vi "Measurement_input_panel.vi"(0 "OK":T4, 2 "setup":T5, 5 "Setup filename":string) -> (11 "Setup filename out":string, 12 "Analysis Info cluster":T8[](array[typedef])=[{"Colour"=0, "Inst type"=enum."Pitot-static tube", "Inst name"="Manometer voltage", "Symbol"="U", "Code name"="", "Extra Info"="U", "Inst Array"=enum."PWA", "Extra Titles"=[], "Extra Values"=[], "U"=0.0, "u^2"=0.0, "u^3"=0.0, "u^4"=0.0, "Skew_u"=0.0, "Kurt_u"=0.0, "Sd Error in Mean"=0.0, "% u'/U"=0.0, "X"=0.0, "Y"=0.0, "Z"=0.0, "Timescale integral to 25%"=0.0, "Sd Error in Variance"=0.0, "Calib File"=path "", "Calib Constants"=[], "Output Position"=FALSE, "Full Stats"=FALSE, "Av Sampling Rate"=0.0, "Av No of Samples"=0.0, "Total Meas Time (s)"=0.0, "ADAM Ch Name"=""}, {"Colour"=0, "Inst type"=enum."Pitot-static tube", "Inst name"="Manometer voltage", "Symbol"="U", "Code name"="", "Extra Info"="U", "Inst Array"=enum."PWA", "Extra Titles"=[], "Extra Values"=[], "U"=0.0, "u^2"=0.0, "u^3"=0.0, "u^4"=0.0, "Skew_u"=0.0, "Kurt_u"=0.0, "Sd Error in Mean"=0.0, "% u'/U"=0.0, "X"=0.0, "Y"=0.0, "Z"=0.0, "Timescale integral to 25%"=0.0, "Sd Error in Variance"=0.0, "Calib File"=path "", "Calib Constants"=[], "Output Position"=FALSE, "Full Stats"=FALSE, "Av Sampling Rate"=0.0, "Av No of Samples"=0.0, "Total Meas Time (s)"=0.0, "ADAM Ch Name"=""}, {"Colour"=0, "Inst type"=enum."Pitot-static tube", "Inst name"="Manometer voltage", "Symbol"="U", "Code name"="", "Extra Info"="U", "Inst Array"=enum."PWA", "Extra Titles"=[], "Extra Values"=[], "U"=0.0, "u^2"=0.0, "u^3"=0.0, "u^4"=0.0, "Skew_u"=0.0, "Kurt_u"=0.0, "Sd Error in Mean"=0.0, "% u'/U"=0.0, "X"=0.0, "Y"=0.0, "Z"=0.0, "Timescale integral to 25%"=0.0, "Sd Error in Variance"=0.0, "Calib File"=path "", "Calib Constants"=[], "Output Position"=FALSE, "Full Stats"=FALSE, "Av Sampling Rate"=0.0, "Av No of Samples"=0.0, "Total Meas Time (s)"=0.0, "ADAM Ch Name"=""}] {"Sd Error in Variance" format="%.2f"; "Skew_u" format="%.2f"; "% u'/U" format="%.2f"; "Sd Error in Mean" format="%.2f"; "Kurt_u" format="%.2f"; "u^4" format="%.2f"; "u^3" format="%.2f"; "U" format="%.2f"; "u^2" format="%.2f"})   [LabVIEW 2013]
uses:
  Controls/Inst_type.ctl
  Controls/Analysis_info_cluster.ctl
  Controls/Instrument_Array.ctl
  Controls/LDA_Setup.ctl
  Controls/Setup.ctl
  Controls/ok_button.ctl
  Controls/Trigger_Mode.ctl
  Controls/PWA_Data.ctl
  File/Setup_Filetype.ctl
  Controls/Post_Process.ctl
  Controls/App_Global.ctl
  Controls/Ch_and_Spans.ctl
  Globals/Meas_global.vi
  Globals/Trav_pos_global.vi
  Globals/LDA_meas_global_1.vi
  Globals/Preference_global.vi
panel:
  in  "Acquisition Plug in":u16(ring) items=["ADAM_Server_Channels.vi", "DataTranslation.vi", "DT_With_Multiplexer.vi", "LDA_IP.vi", "NI-DAQmx.vi", "Simulate_kernal.vi"]
  in  "Select Duplicate Channels":bool
  in  "PWA Data":T1
  out "Inst type":T2
  in  "Edit temp and Press":bool
  out "Abs Press (mbar)":dbl=1013.0 format="%.1f"
  out "Temp (deg C)":dbl=21.0 format="%.1f"
  in  "Trigger mode":T3
  in  "Select Plug Ins":bool
  in  "Sync Delay Time (ms)":dbl=24.0 format="%.2f"
  out "XW Present?":bool
  out "Read Setup File?":bool
  out "Setup Paths":string[](array[string])
  in  "Select ADAM Channels":bool
  in  "stop":bool
  out "Notes":string
  in  "Setup filename selector":u16(ring) items=["Current_Setup.xls", "Copy of Current_Setup.xls", "thermistor-rake.xls", "Current_Setup.xls", "thermistor-rake.xls"]
  in  "Synchronise Analogue channels with LDA":bool
  in  "LDA set up":T6={"dimensions"=enum."2D", "Analogue Freq Multiplier"=0.1} {"Analogue Freq Multiplier" min=0.1 max=100.0 format="%_5g"}
  in  "LDA data":enum16{"No LDA data", "Take LDA data"}(ring)=enum."Take LDA data"
  in  "Cross wire":T7(ring)
  in  "No of Analogue inst":i32=1
  in  "Ch & spans choices":T10(array[cluster]) {"D" format="%.2f"; "Ch No" min=0; "low limit" min=-10 max=10 format="%.2f"; "high limit" min=-10 max=10 format="%.2f"}
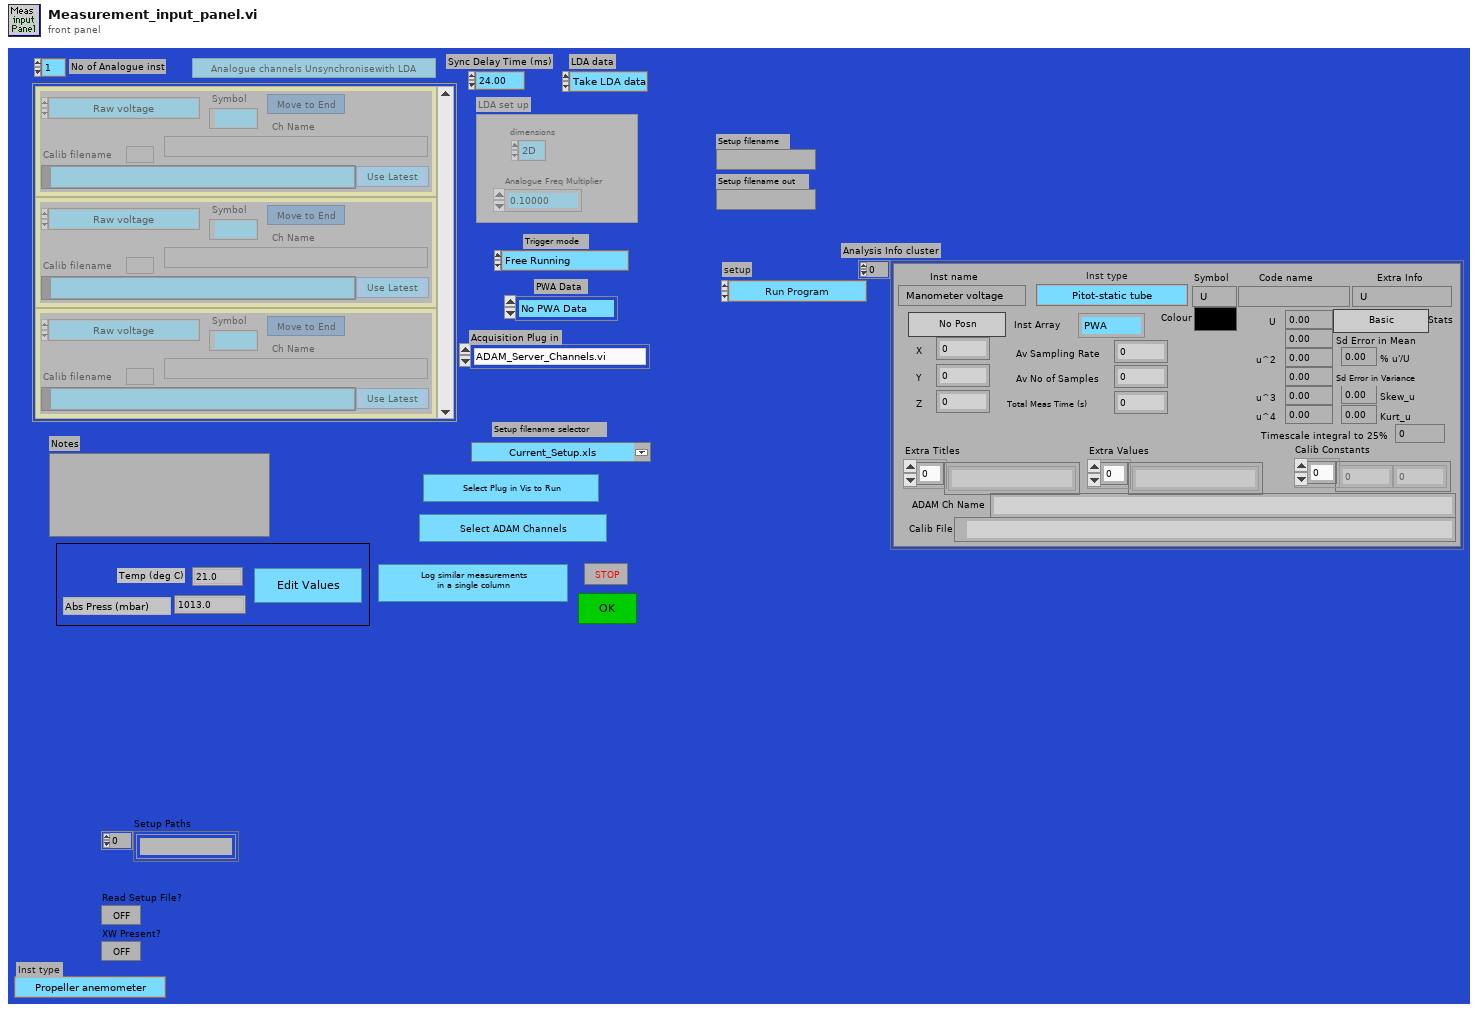
[diagram p1: front panel]
types:
  T1 = typedef "PWA_Data.ctl" = enum16{"No PWA Data", "One Ch PWA"}
  T2 = typedef "Inst_type.ctl" = enum16{"Propeller anemometer", "Raw voltage", "Pressure Transducer", "Pitot-static tube", "Preston tube", "Hot wire", "Cross wire 1", "Cross wire 2", "Generic Linear", "Generic Polynomial", "Generic BackPoly", "Fast FID", "Thermocouple", "Cold wire", "Pulsed Wire", "LDA Vel", "LDA Tran time", "LDA Arr time"}
  T3 = typedef "Trigger_Mode.ctl" = enum16{"Free Running", "Start on Trigger", "Trigger Every Block", "Trigger Every Sample"}
  T4 = typedef "ok_button.ctl" = bool
  T5 = typedef "Setup.ctl" = enum16{"Run Program", "Show Setup", "Save Current Setup", "Setup Front Panel"}
  T6 = typedef "LDA_Setup.ctl" = cluster{"dimensions":enum16{"1D", "2D"}, "Analogue Freq Multiplier":dbl}
  T7 = enum16{"2nd component as calculated", "2nd component multipled by -1"}
  T8 = typedef "Analysis_info_cluster.ctl" = cluster{"Colour":u32, "Inst type":T2, "Inst name":string, "Symbol":string, "Code name":string, "Extra Info":string, "Inst Array":T9, "Extra Titles":string[], "Extra Values":string[], "U":dbl, "u^2":dbl, "u^3":dbl, "u^4":dbl, "Skew_u":dbl, "Kurt_u":dbl, "Sd Error in Mean":dbl, "% u'/U":dbl, "X":dbl, "Y":dbl, "Z":dbl, "Timescale integral to 25%":dbl, "Sd Error in Variance":dbl, "Calib File":path, "Calib Constants":dbl[], "Output Position":bool, "Full Stats":bool, "Av Sampling Rate":dbl, "Av No of Samples":dbl, "Total Meas Time (s)":dbl, "ADAM Ch Name":string}
  T9 = typedef "Instrument_Array.ctl" = enum16{"PWA", "LDA", "Analogue"}
  T10 = cluster{"high limit":sgl, "low limit":sgl, "Ch No":i16, "Calib filename":path, "Inst type":T2, "Symbol":string, "Move channel":bool, "Use Latest":bool, "D":dbl, "Ch Name":string}[]
  T11 = typedef "Post_Process.ctl" = enum16{"Take New Data", "Post Process Raw Data File"}
  T12 = typedef "Setup_Filetype.ctl" = enum16{"Measurement Setups", "Calibration Setups", "General", "Results File Plotter Setups", "Speed Calib Tweaks"}
  T13 = typedef "App_Global.ctl" = enum16{"Read Global", "Write to Global", "Initialise Array"}
  T14 = typedef "Ch_and_Spans.ctl" = cluster{"high limit (10V)":sgl, "low limit (-10V)":sgl, "Ch No":i16, "Var name":string, "Use Latest Calib":bool}
  T15 = enum16{"Zero or one", "One", "Zero or more", "One or more"}
  T16 = typedef "Traverse_cluster.ctl" = cluster{"Start X":dbl, "Start Y":dbl, "Start Z":dbl, "End X":dbl, "End Y":dbl, "End Z":dbl, "No. of pts.":i32, "Spacing":T17, "Filename":path, "Tunnel Speed":dbl, "Averaging time (min)":dbl, "Extra Commands":string, "Specific Arguments":string, "Emission Rate (l/min)":dbl, "Trace Gas Concentration (%)":dbl, "Density Ratio":string, "Comments":string, "Row No":i32, "Row Type Selector":T18, "Completion time":string, "Row Duration (mins)":dbl, "No. of Valid pts.":i32, "Meas Setup File":string}
  T17 = typedef "Spacing.ctl" = enum16{"Linear", "Log", "Gauss", "Specified", "N/A"}
  T18 = typedef "Multi_run_mode.ctl" = enum16{"Move Traverse Only", "Set Tunnel Speed Only", "Set Source Only", "Set Measurement Conditions", "Single Measurement", "Vertical Profile", "Lateral Profile", "Longitudinal Profile", "Explore Volume", "Multi-Axis Profile", "Auto Calibrate", "Meas Fast FID Bkgnd", "Check Beam Power", "Scanning Valve Measurement", "Run VI Named:", "Set ADAM Ch", "Wait (minutes)", "Send Message", "Synchronize With:", "Fall Back to this Row", "Turn Off Row Repeating", "Blank Row", "Traverse 3D Volume"}
  T19 = cluster{"high limit (10V)":sgl, "low limit (-10V)":sgl, "Ch No":i16, "Calib filename":path, "Inst type":T2, "Symbol":string, "Move channel":bool, "Use Latest":bool, "D":dbl, "Ch Name":string}[]
  T20 = cluster{"high limit":sgl, "low limit":sgl, "Ch No":i16, "Calib filename":path, "Inst type":T2, "Symbol":string, "Move channel":bool, "Use Latest":bool, "D":dbl, "Ch Name":string}
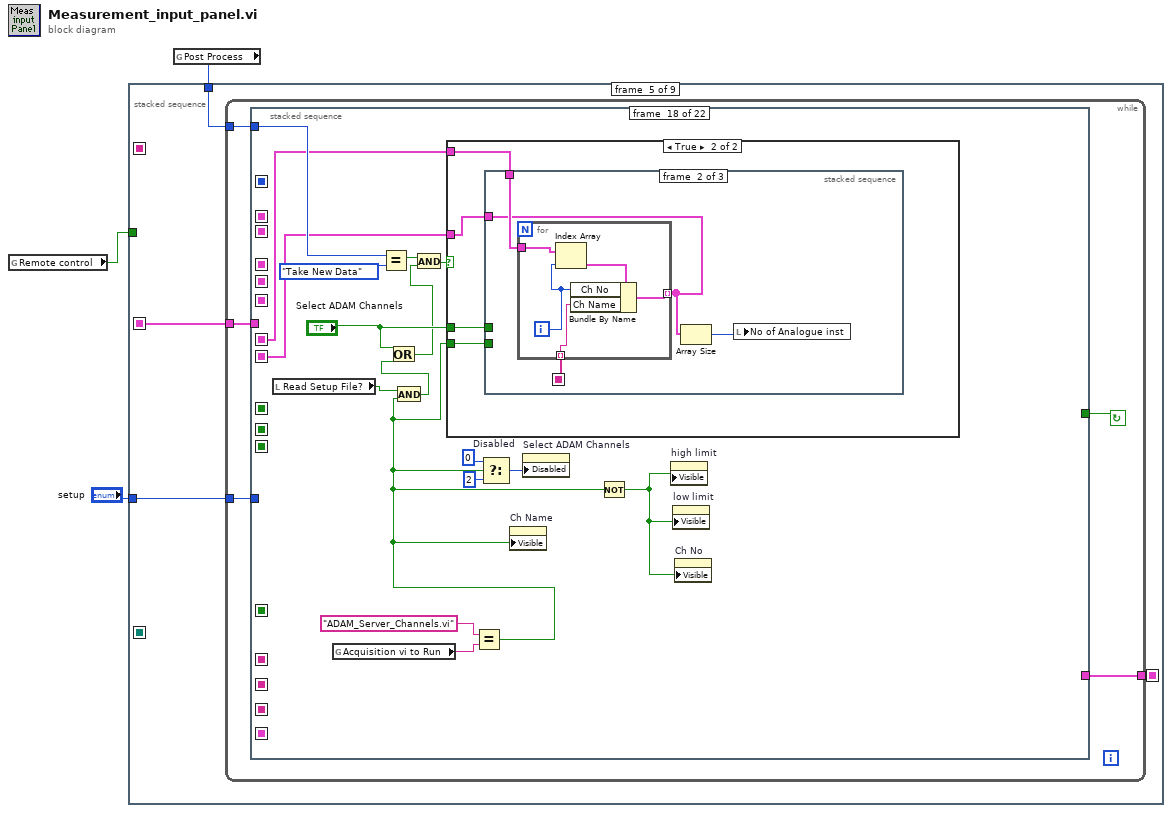
[diagram p0: block diagram]
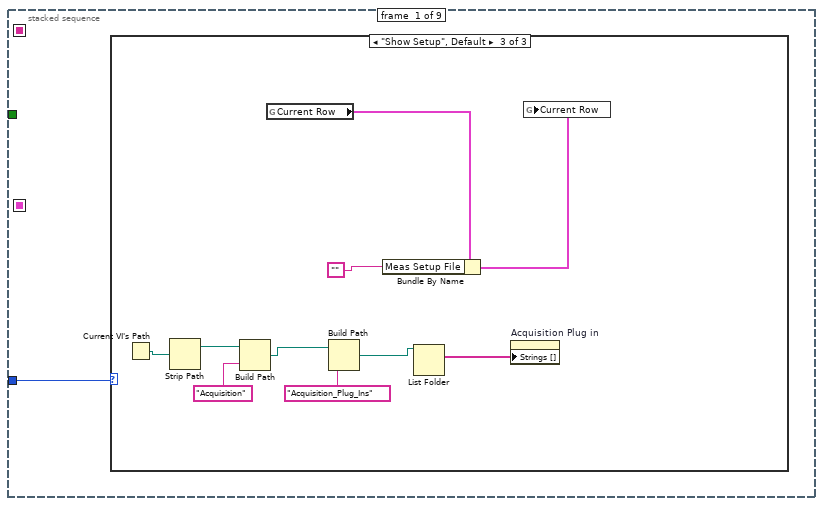
[diagram p2: hidden frame]
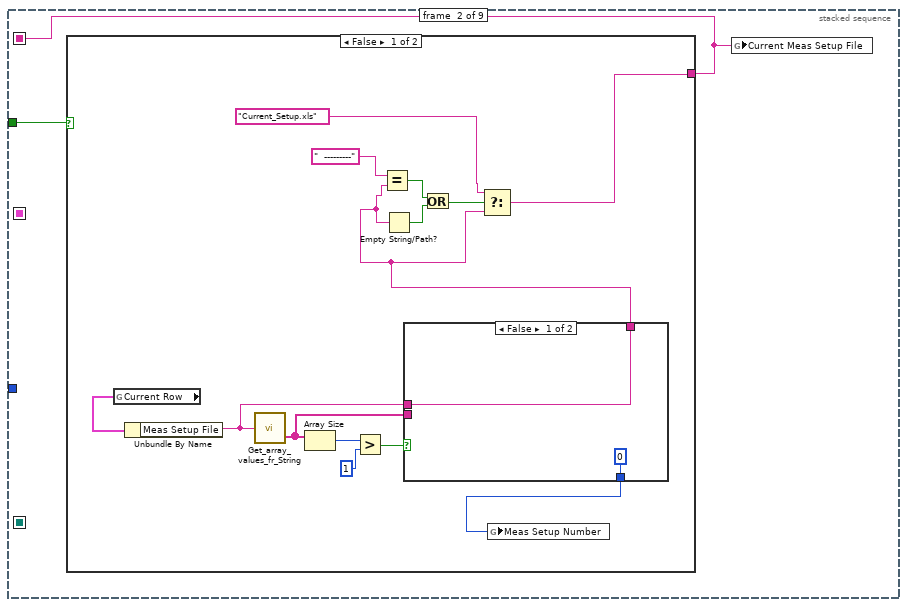
[diagram p5: hidden frame]
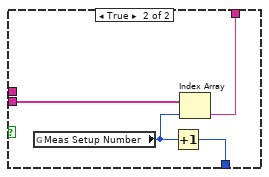
[diagram p6: hidden frame]
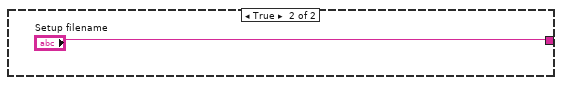
[diagram p7: hidden frame]
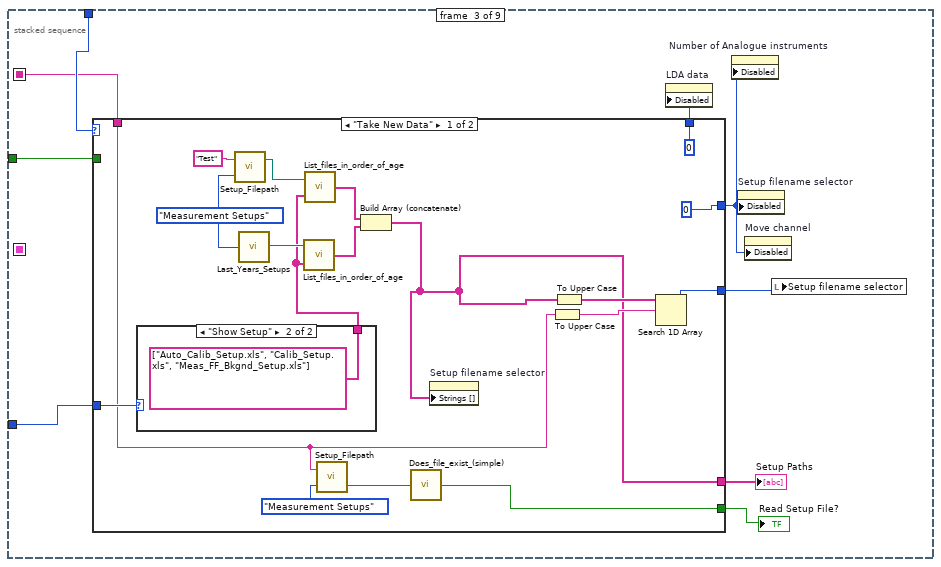
[diagram p8: hidden frame]
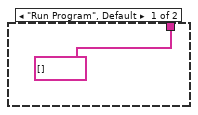
[diagram p9: hidden frame]
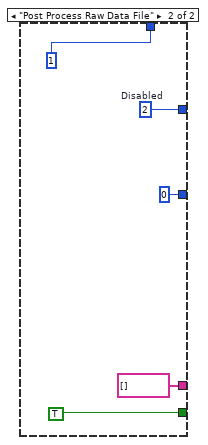
[diagram p10: hidden frame]
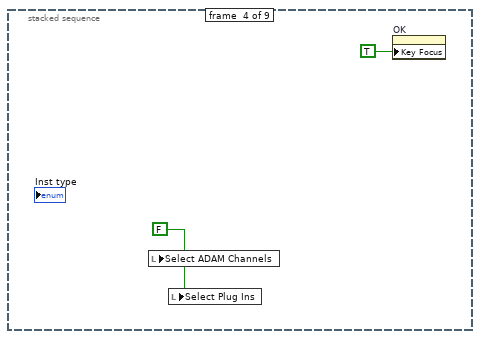
[diagram p11: hidden frame]
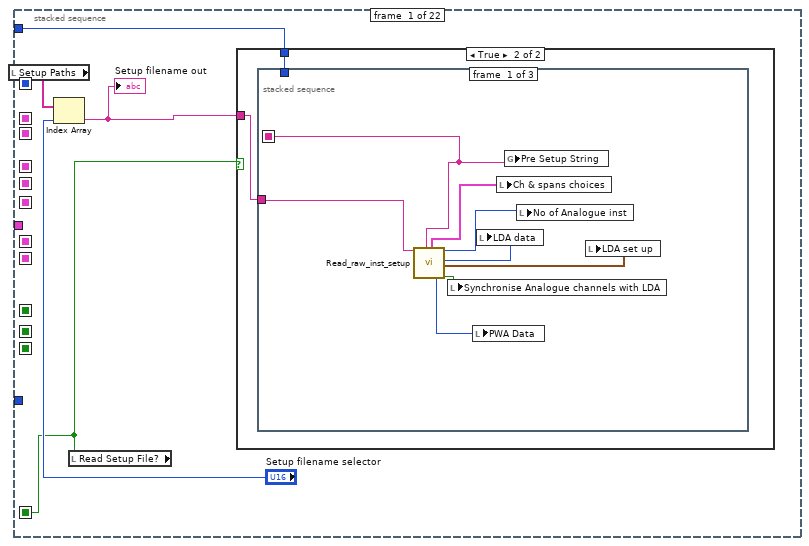
[diagram p12: hidden frame]
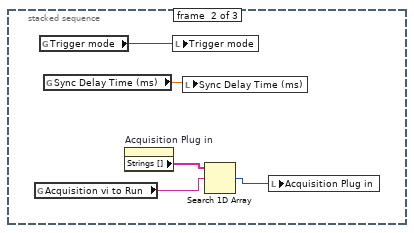
[diagram p14: hidden frame]
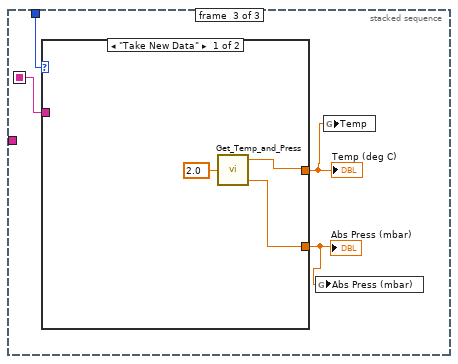
[diagram p15: hidden frame]
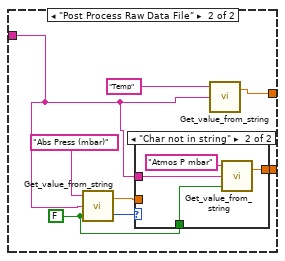
[diagram p16: hidden frame]
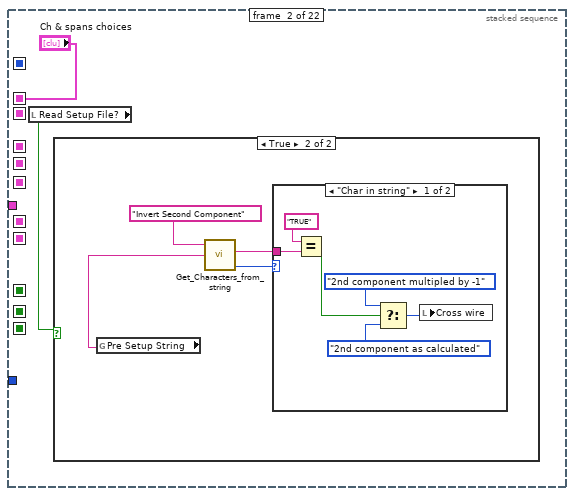
[diagram p18: hidden frame]
diagram:
  n1 = global read "Meas_global.vi" "Remote control"() -> (w1:bool)
  n2 = global read "Meas_global.vi" "Post Process"() -> (w3:T11)
  n3 = stacked-sequence {
    seq-local: [_ _ _ _ w77 _ _ _ _] -> [_ _ _ _ _ _ w694 w795 _]
    seq-local: [_ w15 _ _ _ _ _ _ _] -> [_ _ w38 _ _ _ w693 _ _]
    seq-local: [_ _ _ _ w74 _ _ _ _] -> [_ _ _ _ _ _ _ _ w847]
    seq-local: [_ _ _ _ _ _ _ w794 _] -> [_ _ _ _ _ _ _ _ w846]
    tunnel: w3 -> [_ _ w46 _ w76 _ _ w796 _]
    tunnel: "setup" -> [w4 _ w40 _ w75 _ w695 _ _]
    tunnel: w1 -> [_ w16 w39 _ _ _ _ _ _]
    frame #0 {
      n4 = case shown="\"Show Setup\", Default" w4 {
        frame "Run Program" {
        }
        frame "Setup Front Panel" {
        }
        frame "Show Setup", Default {
          n5 = Current VI's Path() -> (path=w11:path)
          n6 = Strip Path(path=w11) -> (stripped path=w10:path)  [unwired: 1 out]
          n7 = Build Path(base path=w10, name or relative path="Acquisition") -> (appended path=w7:path)
          n8 = global read "Trav_pos_global.vi" "Current Row"() -> (w14:T16)
          n9 = Build Path(base path=w7, name or relative path="Acquisition_Plug_Ins") -> (appended path=w6:path)
          n10 = Bundle By Name(cluster=w14, "Meas Setup File"="") -> (w13:T16)
          n11 = List Folder(path=w6) -> (filenames=w5:string[])  [unwired: 3 in, 3 out]
          n12 = property on="Acquisition Plug in" class="Ring (strict)"("Strings []"=w5) -> ()  [unwired: 2 in, 2 out]
          n13 = global write "Trav_pos_global.vi" "Current Row"(w13) -> ()
        }
      }
    }
    frame #1 {
      n14 = case shown="False" w16 {
        tunnel: [w29 "Setup filename"] -> w15
        frame False {
          n15 = global read "Trav_pos_global.vi" "Current Row"() -> (w25:T16)
          n16 = Unbundle By Name(w25) -> ("Meas Setup File"=w19:string)
          n17 = call "Get_array_values_fr_String.vi"("String Value"=w19) -> ("String array"=w18:string[])  [unwired: 1 out]
          n18 = Array Size(array=w18) -> (size(s)=w23:i32)
          n19 = Greater?(x=w23, y=1) -> (0:w21:bool)
          n20 = case shown="False" w21 {
            tunnel: [w32 w35] -> w20
            tunnel: w19 -> [w32 _]
            tunnel: w18 -> [_ w36]
            tunnel: [0 w33] -> w17
            frame False {
            }
            frame True {
              n21 = global read "Trav_pos_global.vi" "Meas Setup Number"() -> (w34:i32)
              n22 = Increment(x=w34) -> (x+1=w33:i32)
              n23 = Index Array(array=w36, index=w34) -> (element=w35:string)
            }
          }
          n24 = Equal?(x="  ---------" ("f"), y=w20) -> (x = y?=w28:bool)
          n25 = Empty String/Path?(string/path=w20) -> (empty?=w27:bool)
          n26 = Or(x=w28, y=w27) -> (x .or. y?=w24:bool)
          n27 = Select(t="Current_Setup.xls", s=w24, f=w20) -> (s? t:f=w29:string)
          n28 = global write "Trav_pos_global.vi" "Meas Setup Number"(w17) -> ()
        }
        frame True {
        }
      }
      n29 = global write "Trav_pos_global.vi" "Current Meas Setup File"(w15) -> ()
    }
    frame #2 {
      n30 = case shown="\"Take New Data\"" w46 {
        tunnel: [w47 string[] []] -> w42
        tunnel: [w60 TRUE ("exists")] -> w41
        tunnel: [u8 0 ("Disabled") w68] -> w43
        tunnel: [u8 0 ("Disabled") u8 1 ("Disabled")] -> w45
        tunnel: w38 -> [w56 _]
        tunnel: [w63 0 ("index of element")] -> w44
        tunnel: w40 -> [w58 _]
        tunnel: w39 -> [_ _]
        frame "Take New Data" {
          w50 = Setup_Filetype."Measurement Setups" ("Setup File Type")
          n31 = case shown="\"Show Setup\"" w58 {
            tunnel: [string[] [] ("file names") string[] ["Auto_Calib_Setup.xls", "Calib_Setup.xls", "Meas_FF_Bkgnd_Setup.xls"] ("file names")] -> w48
            frame "Run Program", Default {
            }
            frame "Show Setup" {
            }
          }
          n32 = call "Setup_Filepath.vi"("Setup File Type"=w50, "Filename in"="Test") -> ("Directory"=w51:path)  [unwired: 1 out]
          n33 = call "Last_Years_Setups.vi"("Setup File Type"=w50) -> ("Directory"=w49:path)
          n34 = call "List_files_in_order_of_age.vi"("Files to Hide"=w48, "Folder"=w49) -> ("file names"=w53:string[])
          n35 = call "List_files_in_order_of_age.vi"("Files to Hide"=w48, "Folder"=w51) -> ("file names"=w52:string[])
          n36 = call "Setup_Filepath.vi"("Setup File Type"=Setup_Filetype."Measurement Setups", "Filename in"=w56) -> ("Filename Out"=w55:path)  [unwired: 1 out]
          n37 = Build Array (concatenate)(w52, w53) -> (w47:string[])
          n38 = call "Does_file_exist_(simple).vi"("Pathname"=w55) -> ("exists?"=w60:bool)
          n39 = property on="Setup filename selector" class="Ring (strict)"("Strings []"=w47) -> ()  [unwired: 2 in, 2 out]
          n40 = To Upper Case(1:w56) -> (0:w61:string)
          n41 = To Upper Case(1:w47) -> (0:w62:string[])
          n42 = Search 1D Array(1D array=w62, element=w61) -> (index of element=w63:i32)  [unwired: 1 out]
        }
        frame "Post Process Raw Data File" {
          w68 = u8 2  # Disabled
        }
      }
      "Setup Paths" <- w42
      "Read Setup File?" <- w41
      n43 = property on="LDA data" class="Enum (strict)"("Disabled"=w45) -> ()  [unwired: 2 in, 2 out]
      n44 = property on="Number of Analogue instruments" class="DigNum (strict)"("Disabled"=w43) -> ()  [unwired: 2 in, 2 out]
      n45 = property on="Setup filename selector" class="Ring (strict)"("Disabled"=w43) -> ()  [unwired: 2 in, 2 out]
      n46 = property on="Move channel" class="Bool (strict)"("Disabled"=w43) -> ()  [unwired: 2 in, 2 out]
      n47 = local write "Setup filename selector"(w44) -> ()
    }
    frame #3 {
      w73 = FALSE ("Select Local ADAM Channels")
      n48 = local write "Select ADAM Channels"(w73) -> ()
      n49 = local write "Select Plug Ins"(w73) -> ()
      n50 = property on="OK" class="Bool"("Key Focus"=TRUE) -> ()  [unwired: 2 in, 2 out]
    }
    frame #4 {
      n51 = while {
        tunnel: w75 -> [w79]
        tunnel: w76 -> [w80]
        tunnel: [w82] -> w77
        tunnel: [w78] -> w74
        stop <- w81 continue-if-true
        n52 = stacked-sequence {
          seq-local: [_ _ _ _ _ _ _ _ w198 _ _ _ _ _ _ _ _ _ _ _ _ _] -> [_ _ _ _ _ _ _ _ _ _ w261 w306 w351 _ _ _ _ _ _ _ _ _]
          seq-local: [_ "Ch & spans choices" _ _ _ _ _ _ _ _ _ _ _ _ _ _ _ _ _ _ _ _] -> [_ _ _ _ _ w160 _ w194 w199 _ _ _ _ _ _ _ _ _ w579 _ _ _]
          seq-local: [_ _ _ _ _ w165 _ _ _ _ _ _ _ _ _ _ _ _ _ _ _ _] -> [_ _ _ _ _ _ _ _ w200 _ _ _ _ _ _ _ _ _ _ _ _ _]
          seq-local: [_ _ _ _ _ _ _ _ _ _ w263 _ _ _ _ _ _ _ _ _ _ _] -> [_ _ _ _ _ _ _ _ _ _ _ w308 _ _ _ _ _ _ _ _ _ w659]
          seq-local: [_ _ _ _ _ _ _ _ _ _ _ _ _ w384 _ _ _ _ _ _ _ _] -> [_ _ _ _ _ _ _ _ _ _ _ _ _ _ w403 _ _ _ _ _ _ _]
          seq-local: [_ _ _ _ _ _ _ _ _ _ _ _ _ _ w399 _ _ _ _ _ _ _] -> [_ _ _ _ _ _ _ _ _ _ _ _ _ _ _ w427 w493 _ _ _ w635 w660]
          seq-local: [_ _ _ _ _ _ _ _ _ _ _ w312 _ _ _ _ _ _ _ _ _ _] -> [_ _ _ _ _ _ _ _ _ _ _ _ _ w381 _ _ _ _ _ _ _ _]
          seq-local: [_ _ _ _ _ _ _ _ _ _ _ _ w355 _ _ _ _ _ _ _ _ _] -> [_ _ _ _ _ _ _ _ _ _ _ _ _ w380 _ _ _ _ _ _ _ _]
          seq-local: [_ _ _ _ _ _ _ _ _ w258 _ _ _ _ _ _ _ _ _ _ _ _] -> [_ _ _ _ _ _ _ _ _ _ w262 w309 _ _ _ _ _ _ _ _ _ w658]
          seq-local: [_ _ _ _ _ _ _ _ _ _ _ _ _ _ _ w426 _ _ _ _ _ _] -> [_ _ _ _ _ _ _ _ _ _ _ _ _ _ _ _ w496 _ _ _ _ _]
          seq-local: [_ _ _ _ _ _ _ _ _ _ _ _ _ _ _ w425 _ _ _ _ _ _] -> [_ _ _ _ _ _ _ _ _ _ _ _ _ _ _ _ w495 _ _ _ _ _]
          seq-local: [_ _ _ _ _ _ _ _ _ _ _ _ _ _ _ w424 _ _ _ _ _ _] -> [_ _ _ _ _ _ _ _ _ _ _ _ _ _ _ _ w494 _ _ _ _ _]
          seq-local: [_ _ _ _ _ _ _ _ _ _ _ _ _ _ _ _ w492 _ _ _ _ _] -> [_ _ _ _ _ _ _ _ _ _ _ _ _ _ _ _ _ _ _ w585 _ _]
          seq-local: [_ _ _ _ _ _ _ _ _ _ _ _ _ _ _ _ w490 _ _ _ _ _] -> [_ _ _ _ _ _ _ _ _ _ _ _ _ _ _ _ _ w540 _ _ _ _]
          seq-local: [w83 _ _ _ _ _ _ _ _ _ _ _ _ _ _ _ _ _ _ _ _ _] -> [_ _ _ _ _ _ _ _ _ _ _ _ _ _ _ _ w489 _ _ _ _ _]
          seq-local: [_ _ _ _ _ _ _ _ _ _ _ _ _ _ _ _ _ w539 _ _ _ _] -> [_ _ _ _ _ _ _ _ _ _ _ _ _ _ _ _ _ _ w580 _ _ _]
          tunnel: [_ _ _ _ _ _ _ _ _ _ _ _ _ _ w399 _ _ _ _ _ _ _] -> w82
          tunnel: [_ _ _ _ _ _ _ _ _ _ _ w310 _ _ _ _ _ _ _ _ _ _] -> w81
          tunnel: w80 -> [w85 _ _ w139 _ _ _ _ _ w259 _ w307 _ w383 _ _ _ w551 _ _ w636 _]
          tunnel: w79 -> [_ _ w135 _ w146 _ _ _ _ _ _ _ _ w382 _ _ _ _ _ w587 _ _]
          tunnel: [_ _ _ _ _ _ _ _ _ _ _ _ _ _ _ _ w492 _ _ _ _ _] -> w78
          frame #0 {
            n53 = local read "Setup Paths"() -> (w87:string[])
            n54 = Index Array(array=w87, index="Setup filename selector") -> (element=w84:string)
            "Setup filename out" <- w84
            n55 = local read "Read Setup File?"() -> (w83:bool)
            n56 = case shown="True" w83 {
              tunnel: w84 -> [_ w89]
              tunnel: w85 -> [_ w88]
              frame False {
              }
              frame True {
                n57 = stacked-sequence {
                  seq-local: [w92 _ _] -> [_ _ w105]
                  tunnel: w89 -> [w94 _ _]
                  tunnel: w88 -> [_ _ w106]
                  frame #0 {
                    n58 = call "Read_raw_inst_setup.vi"("Setup file"=w94) -> ("Setup string"=w92:string, "Ch & spans choices"=w91:T19, "PWA Data"=w90:T1, "Number of Analogue instruments"=w97:i32, "LDA data"=w96:enum16{"No LDA data", "Take LDA data"}, "LDA set up"=w93:T6, "Synchronise Analogue channels with LDA"=w95:bool)  [unwired: 12 out]
                    n59 = local write "Synchronise Analogue channels with LDA"(w95) -> ()
                    n60 = local write "PWA Data"(w90) -> ()
                    n61 = local write "LDA data"(w96) -> ()
                    n62 = local write "Ch & spans choices"(w91) -> ()
                    n63 = global write "Meas_global.vi" "Pre Setup String"(w92) -> ()
                    n64 = local write "No of Analogue inst"(w97) -> ()
                    n65 = local write "LDA set up"(w93) -> ()
                  }
                  frame #1 {
                    n66 = global read "Meas_global.vi" "Acquisition vi to Run"() -> (w99:string)
                    n67 = global read "Meas_global.vi" "Trigger mode"() -> (w101:T3)
                    n68 = global read "LDA_meas_global_1.vi" "Sync Delay Time (ms)"() -> (w102:dbl)
                    n69 = property on="Acquisition Plug in" class="Ring (strict)"() -> ("Strings []"=w100:string[])  [unwired: 2 in, 2 out]
                    n70 = local write "Trigger mode"(w101) -> ()
                    n71 = local write "Sync Delay Time (ms)"(w102) -> ()
                    n72 = Search 1D Array(1D array=w100, element=w99) -> (index of element=w98:i32)  [unwired: 1 in]
                    n73 = local write "Acquisition Plug in"(w98) -> ()
                  }
                  frame #2 {
                    n74 = case shown="\"Take New Data\"" w106 {
                      tunnel: w105 -> [_ w112]
                      tunnel: [w107 w111] -> w103
                      tunnel: [w108 w110] -> w104
                      frame "Take New Data" {
                        n75 = call "Get_Temp_and_Press.vi"("Averaging time (mins)"=2.0) -> ("Abs Press (mbar)"=w107:dbl, "Temperature"=w108:dbl)  [unwired: 3 out]
                      }
                      frame "Post Process Raw Data File" {
                        w114 = FALSE ("Show Dialog?")
                        n76 = call "Get_value_from_string.vi"("Show Dialog?"=w114, "Input string"=w112, "Variable name"="Abs Press (mbar)") -> ("Status"=w116:enum16{"Char in string", "Char not in string"}, "Value"=w115:dbl)
                        n77 = case shown="\"Char not in string\"" w116 {
                          tunnel: [w118 w121] -> w111
                          tunnel: w115 -> [w118 _]
                          tunnel: w114 -> [_ w120]
                          tunnel: w112 -> [_ w119]
                          frame "Char in string" {
                          }
                          frame "Char not in string" {
                            n78 = call "Get_value_from_string.vi"("Show Dialog?"=w120, "Input string"=w119, "Variable name"="Atmos P mbar") -> ("Value"=w121:dbl)  [unwired: 1 out]
                          }
                        }
                        n79 = call "Get_value_from_string.vi"("Input string"=w112, "Variable name"="Temp") -> ("Value"=w110:dbl)  [unwired: 1 in, 1 out]
                      }
                    }
                    "Abs Press (mbar)" <- w103
                    "Temp (deg C)" <- w104
                    n80 = global write "Meas_global.vi" "Abs Press (mbar)"(w103) -> ()
                    n81 = global write "Meas_global.vi" "Temp"(w104) -> ()
                  }
                }
              }
            }
          }
          frame #1 {
            n82 = local read "Read Setup File?"() -> (w124:bool)
            n83 = case shown="True" w124 {
              frame False {
              }
              frame True {
                n84 = global read "Meas_global.vi" "Pre Setup String"() -> (w127:string)
                n85 = call "Get_Characters_from_string.vi"("Input string"=w127, "Variable name"="Invert Second Component") -> ("Status"=w126:enum16{"Char in string", "Char not in string"}, "Value"=w125:string)  [unwired: 1 in]
                n86 = case shown="\"Char in string\"" w126 {
                  tunnel: w125 -> [w134 _]
                  frame "Char in string" {
                    n87 = Equal?(x="TRUE", y=w134) -> (x = y?=w130:bool)
                    n88 = Select(t=T7."2nd component multipled by -1" ("Cross wire/LDA"), s=w130, f=T7."2nd component as calculated" ("Cross wire/LDA")) -> (s? t:f=w132:T7)
                    n89 = local write "Cross wire"(w132) -> ()
                  }
                  frame "Char not in string" {
                  }
                }
              }
            }
          }
          frame #2 {
            n90 = case shown="\"Show Setup\"" w135 {
              frame "Run Program", Default {
              }
              frame "Show Setup" {
                n91 = property on="Acquisition Plug in" class="Ring (strict)"() -> ("Strings []"=w138:string[])  [unwired: 2 in, 2 out]
                n92 = Index Array(array=w138, index="Acquisition Plug in") -> (element=w136:string)
                n93 = global write "Meas_global.vi" "Acquisition vi to Run"(w136) -> ()
              }
            }
          }
          frame #3 {
            n94 = case shown="False" "Edit temp and Press" {
              tunnel: w139 -> [_ w141]
              frame False {
              }
              frame True {
                n95 = case shown="\"Take New Data\"" w141 {
                  frame "Take New Data" {
                    n96 = stacked-sequence {
                      frame #0 {
                        w142 = TRUE  # Wait until done
                        n97 = call "Run_Enter_Temp.vi"("Wait until done"=w142) -> ()  [unwired: 1 out]
                      }
                      frame #1 {
                        n98 = call "Get_Temp_and_Press.vi"("Averaging time (mins)"=2.0) -> ("Abs Press (mbar)"=w143:dbl, "Temperature"=w144:dbl)  [unwired: 3 out]
                        n99 = local write "Temp (deg C)"(w144) -> ()
                        n100 = local write "Abs Press (mbar)"(w143) -> ()
                      }
                    }
                  }
                  frame "Post Process Raw Data File" {
                  }
                }
              }
            }
          }
          frame #4 {
            n101 = case shown="True" "Select Plug Ins" {
              tunnel: w146 -> [_ w148]
              frame False {
              }
              frame True {
                n102 = stacked-sequence {
                  tunnel: w148 -> [w149 _]
                  frame #0 {
                    w153 = TRUE  # Show Panel?
                    n103 = global read "Meas_global.vi" "Pre Setup String"() -> (w152:string)
                    n104 = local write "Select Plug Ins"(FALSE ("Select Local ADAM Channels")) -> ()
                    n105 = call "Choose_Plug_In_to_Run.vi"("setup"=w149, "Show Panel?"=w153, "Setup String In"=w152) -> ("Setup String Out"=w151:string)  [unwired: 1 out]
                    n106 = global write "Meas_global.vi" "Pre Setup String"(w151) -> ()
                  }
                  frame #1 {
                    n107 = Current VI's Path() -> (path=w155:path)
                    n108 = call "Open_Close_Front_Panel.ph.vi"("Front Panel Window:Open"=TRUE, "VI path"=w155) -> ()  [unwired: 2 out]
                  }
                }
              }
            }
          }
          frame #5 {
            n109 = Initialize Array(0) -> (w167:i32[])  [unwired: 1 out]
            n110 = for {
              shift-right: [w174] -> w163
              shift-left: w167 -> [w175]
              tunnel: [w173] -> w161 mode=indexing
              tunnel: w160 -> [w172] mode=indexing
              tunnel: [w170] -> w159 mode=indexing
              n111 = Unbundle By Name(w172) -> ("Inst type"=w169:T2)
              n112 = case shown="\"Cross wire 1\"" w169 {
                tunnel: w175 -> [w179 w183 w185 w189]
                tunnel: [w178 w182 w185 w188] -> w174
                tunnel: [FALSE TRUE FALSE FALSE] -> w173
                frame "Propeller anemometer", Default {
                  n113 = Build Array (concatenate)(w179, 1) -> (w178:i32[])
                }
                frame "Cross wire 1" {
                  n114 = Build Array (concatenate)(w183, 2) -> (w182:i32[])
                }
                frame "Cross wire 2" {
                }
                frame "LDA Vel" {
                  n115 = Build Array (concatenate)(w189, 1) -> (w188:i32[])
                }
              }
              n116 = Equal?(x=w169, y=Inst_type."Preston tube" ("Inst type")) -> (x = y?=w170:bool)
            }
            n117 = Build Array (concatenate)(w163, 1) -> (w162:i32[])
            n118 = Array Subset(array=w162, length="No of Analogue inst") -> (w166:i32[])  [unwired: 1 in]
            n119 = Add Array Elements(numeric array=w166) -> (sum=w165:i32)
            n120 = Or Array Elements(Boolean array=w161) -> (logical OR=→"XW Present?":bool)
            n121 = Or Array Elements(Boolean array=w159) -> (logical OR=w157:bool)
            n122 = property on="D" class="DigNum (strict)"("Visible"=w157) -> ()  [unwired: 2 in, 2 out]
          }
          frame #6 {
            "Notes" <- ""
          }
          frame #7 {
            n123 = Array Size(array=w194) -> (size(s)=w193:i32)
            n124 = Not Equal To 0?(x=w193) -> (x != 0?=w192:bool)
            n125 = case shown="True" w192 {
              tunnel: [enum16{"No Analogue data", "Take Analogue data"}."No Analogue data" ("Analogue data") enum16{"No Analogue data", "Take Analogue data"}."Take Analogue data" ("Analogue data")] -> w191
              frame False {
              }
              frame True {
              }
            }
            n126 = global write "Meas_global.vi" "Analogue data"(w191) -> ()
          }
          frame #8 {
            n127 = Index Array(array=w199, index=0) -> (element=w204:T20)
            n128 = Initialize Array(w204) -> (w202:T10)  [unwired: 1 out]
            n129 = Build Array (concatenate)(w199, w204) -> (w203:T10)
            n130 = for {
              N: w200 -> [_]
              tunnel: w203 -> [w212] mode=indexing
              shift-right: [w213] -> w198
              shift-left: w202 -> [w207]
              tunnel: Inst_type."Cross wire 2" ("Inst type") -> [w205]
              shift-right: [w211] -> _
              shift-left: _ -> [w210]
              tunnel: w203 -> [w209]
              n131 = Unbundle By Name(w212) -> ("Inst type"=w211:T2)
              n132 = Array Size(array=w207) -> (size(s)=w206:i32)
              n133 = Increment(x=w206) -> (x+1=w208:i32)
              n134 = case shown="\"Cross wire 2\"" w211 {
                tunnel: [w222 w243 w255] -> w213
                tunnel: w207 -> [w223 w245 w257]
                tunnel: w212 -> [w219 w246 w256]
                tunnel: w205 -> [w221 w250 _]
                tunnel: w210 -> [_ w249 _]
                tunnel: w209 -> [w226 _ _]
                tunnel: w208 -> [w225 _ _]
                frame "Cross wire 1" {
                  n135 = Index Array(array=w226, index=w225) -> (element=w220:T20)
                  n136 = Unbundle By Name(w220) -> ("Inst type"=w224:T2, "high limit"=w217:sgl, "low limit"=w216:sgl, "Ch No"=w215:i16, "Symbol"=w214:string)
                  n137 = Unbundle By Name(w219) -> ("Calib filename"=w218:path)
                  n138 = case shown="\"Generic Linear\", Default" w224 {
                    tunnel: w223 -> [w236 w242]
                    tunnel: [w235 w241] -> w222
                    tunnel: w221 -> [w228 w237]
                    tunnel: w218 -> [w234 w240]
                    tunnel: w219 -> [w232 w238]
                    tunnel: w220 -> [_ _]
                    tunnel: w217 -> [w231 _]
                    tunnel: w216 -> [w230 _]
                    tunnel: w215 -> [w229 _]
                    tunnel: w214 -> [w227 _]
                    frame "Cross wire 2" {
                      n139 = Bundle By Name(cluster=w232, "Calib filename"=w234, "Inst type"=w228, "high limit"=w231, "low limit"=w230, "Ch No"=w229, "Symbol"=w227) -> (w233:T20)
                      n140 = Build Array (concatenate)(w236, w232, w233) -> (w235:T10)
                    }
                    frame "Generic Linear", Default {
                      n141 = Bundle By Name(cluster=w238, "Calib filename"=w240, "Inst type"=w237) -> (w239:T20)
                      n142 = Build Array (concatenate)(w242, w238, w239) -> (w241:T10)
                    }
                  }
                }
                frame "Cross wire 2" {
                  n143 = Decrement(x=w250) -> (x-1=w248:T2)
                  n144 = Equal?(x=w248, y=w249) -> (x = y?=w247:bool)
                  n145 = Bundle By Name(cluster=w246, "Inst type"=w248) -> (w244:T20)
                  n146 = case shown="False" w247 {
                    tunnel: w246 -> [_ _]
                    tunnel: w245 -> [w253 w254]
                    tunnel: w244 -> [w252 _]
                    tunnel: [w251 w254] -> w243
                    frame False {
                      n147 = Build Array (concatenate)(w253, w252) -> (w251:T10)
                    }
                    frame True {
                    }
                  }
                }
                frame "Generic Linear", Default {
                  n148 = Build Array (concatenate)(w257, w256) -> (w255:T10)
                }
              }
            }
          }
          frame #9 {
            n149 = Equal?(x=w259, y=Post_Process."Take New Data" ("Post Process")) -> (x = y?=w258:bool)
          }
          frame #10 {
            n150 = case shown="True" "OK" {
              tunnel: w261 -> [_ w278]
              tunnel: [FALSE w277] -> w263
              tunnel: w262 -> [_ w266]
              frame False {
              }
              frame True {
                n151 = for {
                  tunnel: w278 -> [w290] mode=indexing
                  tunnel: [w288] -> w272 mode=indexing
                  tunnel: [w284] -> w276 mode=indexing
                  n152 = Unbundle By Name(w290) -> ("high limit"=w293:sgl, "low limit"=w292:sgl, "Ch No"=w289:i16, "Inst type"=w287:T2, "Symbol"=w286:string)
                  n153 = Number To Decimal String(number=w287) -> (decimal integer string=w285:string)  [unwired: 1 out]
                  n154 = Concatenate Strings(w285, w286) -> (w284:string)
                  n155 = Greater Or Equal?(x=w293, y=w292) -> (x >= y?=w291:bool)
                  n156 = case shown="\"Propeller anemometer\", Default" w287 {
                    tunnel: w291 -> [w296 _ _ _]
                    tunnel: w289 -> [w295 _ _ _]
                    tunnel: [w294 TRUE TRUE TRUE] -> w288
                    frame "Propeller anemometer", Default {
                      n157 = case shown="True" w296 {
                        tunnel: w295 -> [w299 _]
                        tunnel: [FALSE TRUE] -> w294
                        frame False {
                          n158 = Number To Decimal String(number=w299) -> (decimal integer string=w298:string)  [unwired: 1 out]
                          n159 = Concatenate Strings("Error in input limits for Channel No ", w298) -> (w300:string)
                          n160 = One Button Dialog(message=w300) -> ()  [unwired: 2 out]
                        }
                        frame True {
                        }
                      }
                    }
                    frame "LDA Vel" {
                    }
                    frame "LDA Tran time" {
                    }
                    frame "LDA Arr time" {
                    }
                  }
                }
                n161 = call "Analyse_string_array.vi"("String array"=w276) -> ("Frequency"=w275:i32[])  [unwired: 2 out]
                n162 = global read "Meas_global.vi" "Remote control"() -> (w267:bool)
                n163 = Greater?(x=w275, y=1) -> (0:w273:bool[])
                n164 = Or Array Elements(Boolean array=w273) -> (logical OR=w269:bool)
                n165 = Compound Arithmetic op=AND(invert w267, w269, w266) -> (w268:bool)
                n166 = case shown="True" w268 {
                  tunnel: [TRUE FALSE] -> w271
                  frame False {
                  }
                  frame True {
                    n167 = Current VI's Path() -> (path=w281:path)
                    n168 = call "Open_Close_Front_Panel.ph.vi"("Front Panel Window:Open"=TRUE, "VI path"=w281) -> ()  [unwired: 2 out]
                    n169 = One Button Dialog(message="Non Unique symbol names") -> ()  [unwired: 2 out]
                  }
                }
                n170 = Build Array (concatenate)(w272, w271) -> (w270:bool[])
                n171 = And Array Elements(Boolean array=w270) -> (logical AND=w277:bool)
              }
            }
          }
          frame #11 {
            n172 = And(x=w309, y=w308) -> (x .and. y?=w311:bool)
            n173 = case shown="True" w311 {
              tunnel: w306 -> [_ w319]
              tunnel: [FALSE w318] -> w312
              tunnel: [w313 w317] -> w310
              tunnel: w308 -> [w314 _]
              tunnel: w307 -> [_ _]
              frame False {
                n174 = Not(x=w314) -> (.not. x?=w313:bool)
              }
              frame True {
                n175 = for {
                  shift-right: [w338] -> _
                  shift-left: i16[] [] -> [w337]
                  tunnel: w319 -> [w334] mode=indexing
                  tunnel: [w325] -> w320 mode=indexing
                  shift-right: [w333] -> _
                  shift-left: path[] [] -> [w332]
                  n176 = Unbundle By Name(w334) -> ("Ch No"=w335:i16)
                  n177 = Unbundle By Name(w334) -> ("Inst type"=w331:T2, "Calib filename"=w328:path)
                  n178 = Search 1D Array(1D array=w337, element=w335) -> (index of element=w336:i32)  [unwired: 1 out]
                  n179 = Build Array (concatenate)(w337, w335) -> (w338:i16[])
                  n180 = Equal?(x=Inst_type."Fast FID" ("Inst type"), y=w331) -> (x = y?=w324:bool)
                  n181 = case shown="0, Default" w336 {
                    tunnel: w335 -> [w349 _]
                    tunnel: [w345 FALSE ("true")] -> w327
                    frame 0, Default {
                      n182 = Format Into String(format string="The Ch No %d appears more than once", w349) -> (resulting string=w347:string)  [unwired: 2 in, 1 out]
                      n183 = One Button Dialog(message=w347, button name ("OK")="Ok") -> (true=w345:bool)
                    }
                    frame -1 {
                    }
                  }
                  n184 = Search 1D Array(1D array=w332, element=w328) -> (index of element=w329:i32)  [unwired: 1 out]
                  n185 = Greater Or Equal To 0?(x=w329) -> (x >= 0?=w323:bool)
                  n186 = And(x=w324, y=w323) -> (x .and. y?=w322:bool)
                  n187 = case shown="True" w322 {
                    tunnel: [w340 FALSE ("true")] -> w326
                    tunnel: w328 -> [w339 _]
                    frame True {
                      n188 = Format Into String(format string="Calibration file %s is used more than once.", w339) -> (resulting string=w342:string)  [unwired: 2 in, 1 out]
                      n189 = One Button Dialog(message=w342, button name ("OK")="Ok") -> (true=w340:bool)
                    }
                    frame False {
                    }
                  }
                  n190 = Build Array (concatenate)(w332, w328) -> (w333:path[])
                  n191 = Or(x=w327, y=w326) -> (x .or. y?=w325:bool)
                }
                n192 = Or Array Elements(Boolean array=w320) -> (logical OR=w317:bool)
                n193 = Not(x=w317) -> (.not. x?=w318:bool)
              }
            }
          }
          frame #12 {
            n194 = call "Current_Calib_Filenames.vi"("Mode"=App_Global."Read Global") -> ("Calib Filename Out"=w352:path[], "Channel Numbers Out"=w353:i16[])  [unwired: 2 in, 1 out]
            n195 = for {
              tunnel: w351 -> [w366] mode=indexing
              tunnel: w353 -> [w368]
              tunnel: w352 -> [w367]
              tunnel: [w365] -> w355 mode=indexing
              w363 = Inst_type."Cross wire 2"  # Inst type
              n196 = Unbundle By Name(w366) -> ("Inst type"=w358:T2, "Ch No"=w360:i16, "Use Latest"=w361:bool, "Inst type"=w364:T2)
              n197 = Not Equal?(x=w364, y=w363) -> (x != y?=w362:bool)
              n198 = Compound Arithmetic op=AND(w361, w362) -> (w359:bool)
              n199 = Not Equal?(x=Inst_type."Raw voltage" ("Inst type"), y=w358) -> (x != y?=w356:bool)
              n200 = case shown="True" w359 {
                tunnel: w368 -> [_ w379]
                tunnel: w360 -> [_ w378]
                tunnel: w367 -> [_ w376]
                tunnel: w366 -> [w369 w375]
                tunnel: [w369 w374] -> w365
                tunnel: w356 -> [_ w371]
                frame False {
                }
                frame True {
                  n201 = Search 1D Array(1D array=w379, element=w378) -> (index of element=w377:i32)  [unwired: 1 out]
                  n202 = Index Array(array=w376, index=w377) -> (element=w372:path)
                  n203 = Select(t=w372, s=w371, f=path "") -> (s? t:f=w373:path)
                  n204 = Bundle By Name(cluster=w375, "Calib filename"=w373) -> (w374:T20)
                }
              }
            }
          }
          frame #13 {
            n205 = case shown="True" w381 {
              tunnel: w380 -> [w385 w388]
              tunnel: [w385 w387] -> w384
              tunnel: w383 -> [_ _]
              tunnel: w382 -> [_ w386]
              frame False {
              }
              frame True {
                n206 = case shown="\"Run Program\", Default" w386 {
                  tunnel: w388 -> [w390 w398]
                  tunnel: [w389 w398] -> w387
                  frame "Run Program", Default {
                    n207 = for {
                      tunnel: w390 -> [w391] mode=indexing
                      tunnel: [w392] -> w389 mode=indexing
                      n208 = Unbundle By Name(w391) -> ("Calib filename"=w397:path, "Use Latest"=w396:bool, "Ch No"=w395:i16, "Inst type"=w394:T2)
                      n209 = call "Find_calibration_file.vi"("Inst type"=w394, "Ch No"=w395, "Use Latest Calib"=w396, "filename"=w397) -> ("filename out"=w393:path)
                      n210 = Bundle By Name(cluster=w391, "Calib filename"=w393) -> (w392:T20)
                    }
                  }
                  frame "Setup Front Panel" {
                  }
                }
              }
            }
          }
          frame #14 {
            w401 = 0 ("Index")
            n211 = Index Array(array=w403, index=w401) -> (element=w402:T20)
            n212 = Initialize Array(w402, w401) -> (w400:T10)
            n213 = for {
              shift-right: [w411] -> w405
              shift-left: w400 -> [w410]
              shift-right: [w412] -> w406
              shift-left: w400 -> [w414]
              tunnel: w403 -> [w413] mode=indexing
              n214 = Unbundle By Name(w413) -> ("Move channel"=w415:bool)
              n215 = case shown="True" w415 {
                tunnel: w414 -> [w417 w423]
                tunnel: w413 -> [w419 w422]
                tunnel: [w418 w423] -> w412
                tunnel: [w416 w421] -> w411
                tunnel: w410 -> [w416 w420]
                frame False {
                  n216 = Build Array (concatenate)(w417, w419) -> (w418:T10)
                }
                frame True {
                  n217 = Build Array (concatenate)(w420, w422) -> (w421:T10)
                }
              }
            }
            n218 = Build Array (concatenate)(w406, w405) -> (w404:T10)
            n219 = for {
              tunnel: w404 -> [w409] mode=indexing
              tunnel: [w407] -> w399 mode=indexing
              n220 = Bundle By Name(cluster=w409, "Move channel"=FALSE) -> (w407:T20)
            }
          }
          frame #15 {
            n221 = for {
              shift-right: [w433] -> _
              shift-left: string[] [] -> [w434]
              tunnel: [w436] -> w425 mode=indexing
              tunnel: [w430] -> w426 mode=indexing
              tunnel: w427 -> [w432] mode=indexing
              tunnel: [w429] -> w424 mode=indexing
              n222 = Unbundle By Name(w432) -> ("Inst type"=w435:T2)
              n223 = case shown="\"Raw voltage\"" w435 {
                tunnel: [w443 w447 w450 w454 w458 w462 w466 "XW" w473 w478 w481 w485] -> w430
                tunnel: ["U" "P" "U" "U" "tau" "U" "U" "W" "U" "C" "T" "T"] -> w437
                tunnel: w434 -> [w444 w448 w452 w456 w460 w464 w468 w470 w475 w479 w483 w487]
                tunnel: [w442 w446 w451 w455 w459 w463 w467 w470 w474 w477 w482 w486] -> w433
                frame "Propeller anemometer" {
                  w443 = "Prop"
                  n224 = Build Array (concatenate)(w444, w443) -> (w442:string[])
                }
                frame "Pressure Transducer" {
                  w447 = "Mano"
                  n225 = Build Array (concatenate)(w448, w447) -> (w446:string[])
                }
                frame "Raw voltage" {
                  w450 = "RV"
                  n226 = Build Array (concatenate)(w452, w450) -> (w451:string[])
                }
                frame "Pitot-static tube" {
                  w454 = "Pitot"
                  n227 = Build Array (concatenate)(w456, w454) -> (w455:string[])
                }
                frame "Preston tube" {
                  w458 = "Preston"
                  n228 = Build Array (concatenate)(w460, w458) -> (w459:string[])
                }
                frame "Hot wire" {
                  w462 = "HW"
                  n229 = Build Array (concatenate)(w464, w462) -> (w463:string[])
                }
                frame "Cross wire 1" {
                  w466 = "XW"
                  n230 = Build Array (concatenate)(w468, w466) -> (w467:string[])
                }
                frame "Cross wire 2" {
                }
                frame "Generic Linear", Default {
                  w473 = "Gen"
                  n231 = Build Array (concatenate)(w475, w473) -> (w474:string[])
                }
                frame "Fast FID" {
                  w478 = "FF"
                  n232 = Build Array (concatenate)(w479, w478) -> (w477:string[])
                }
                frame "Thermocouple" {
                  w481 = "T"
                  n233 = Build Array (concatenate)(w483, w481) -> (w482:string[])
                }
                frame "Cold wire" {
                  w485 = "CW"
                  n234 = Build Array (concatenate)(w487, w485) -> (w486:string[])
                }
              }
              n235 = call "Analyse_string_array.vi"("String array"=w433) -> ("Unique strings"=w441:string[], "Frequency"=w439:i32[])  [unwired: 1 out]
              n236 = Search 1D Array(1D array=w441, element=w430) -> (index of element=w440:i32)  [unwired: 1 out]
              n237 = Index Array(array=w439, index=w440) -> (element=w431:i32)
              n238 = Number To Decimal String(number=w431) -> (decimal integer string=w429:string)  [unwired: 1 out]
              n239 = Concatenate Strings(w429, w430, ":", w437) -> (w436:string)
            }
          }
          frame #16 {
            w499 = T8 {"Colour"=0, "Inst type"=enum."Pitot-static tube", "Inst name"="Manometer voltage", "Symbol"="U", "Code name"="", "Extra Info"="U", "Inst Array"=enum."PWA", "Extra Titles"=[], "Extra Values"=[], "U"=0.0, "u^2"=0.0, "u^3"=0.0, "u^4"=0.0, "Skew_u"=0.0, "Kurt_u"=0.0, "Sd Error in Mean"=0.0, "% u'/U"=0.0, "X"=0.0, "Y"=0.0, "Z"=0.0, "Timescale integral to 25%"=0.0, "Sd Error in Variance"=0.0, "Calib File"=path "", "Calib Constants"=[], "Output Position"=FALSE, "Full Stats"=FALSE, "Av Sampling Rate"=0.0, "Av No of Samples"=0.0, "Total Meas Time (s)"=0.0, "ADAM Ch Name"=""}  # Analysis info cluster
            n240 = property on="Ch Name" class="Str"() -> ("Visible"=w500:bool)  [unwired: 2 in, 2 out]
            n241 = global read "Meas_global.vi" "Pre Setup String"() -> (w491:string)
            n242 = for {
              tunnel: [w531] -> w498 mode=indexing
              tunnel: w493 -> [w507] mode=indexing
              tunnel: w496 -> [w522] mode=indexing
              tunnel: T14 {"high limit (10V)"=10.0, "low limit (-10V)"=-10.0, "Ch No"=0, "Var name"="", "Use Latest Calib"=FALSE} ("Ch and Spans") -> [w528]
              tunnel: [w527] -> w492 mode=indexing
              tunnel: w495 -> [w510] mode=indexing
              tunnel: w499 -> [w525]
              tunnel: w494 -> [w519] mode=indexing
              tunnel: w500 -> [w502]
              tunnel: w491 -> [w511]
              tunnel: [w506] -> w490 mode=indexing
              tunnel: w489 -> [w501]
              n243 = Unbundle By Name(w507) -> ("Use Latest"=w523:bool, "high limit"=w530:sgl, "low limit"=w529:sgl, "Ch No"=w524:i16, "Inst type"=w517:T2, "Symbol"=w516:string, "D"=w515:dbl, "Ch Name"=w503:string)
              n244 = Empty String/Path?(string/path=w516) -> (empty?=w520:bool)
              n245 = Concatenate Strings(w510, "_ADAM_Ch_Name" ("string")) -> (w508:string)
              n246 = call "Get_Characters_from_string.vi"("Input string"=w511, "Variable name"=w508) -> ("Value"=w505:string)  [unwired: 1 in, 1 out]
              n247 = Select(t=w519, s=w520, f=w516) -> (s? t:f=w518:string)
              n248 = Format Into String(format string="%s (%s)" ("Format String"), w522, w518) -> (resulting string=w513:string)  [unwired: 2 in, 1 out]
              n249 = Select(t=w503, s=w502, f=w513) -> (s? t:f=w512:string)
              n250 = Bundle By Name(cluster=w528, "Use Latest Calib"=w523, "high limit (10V)"=w530, "low limit (-10V)"=w529, "Ch No"=w524, "Var name"=w512) -> (w531:T14)
              n251 = Select(t=w505, s=w501, f=w503) -> (s? t:f=w504:string)
              n252 = case shown="\"Propeller anemometer\", Default" w517 {
                tunnel: [w534 w537] -> w526
                tunnel: w524 -> [w532 _]
                tunnel: w515 -> [_ w535]
                frame "Propeller anemometer", Default {
                  n253 = Format Into String(format string="Ch %d" ("Format String"), w532) -> (resulting string=w534:string)  [unwired: 2 in, 1 out]
                }
                frame "Preston tube" {
                  n254 = Format Into String(format string="D = %.2f" ("Format String"), w535) -> (resulting string=w537:string)  [unwired: 2 in, 1 out]
                }
              }
              n255 = Bundle By Name(cluster=w507, "Ch Name"=w504) -> (w506:T20)
              n256 = Bundle By Name(cluster=w525, "Extra Info"=w526, "Inst type"=w517, "Inst name"=w513, "Symbol"=w518, "Code name"=w510, "Inst Array"=Instrument_Array."Analogue", "ADAM Ch Name"=w504) -> (w527:T8)
            }
            n257 = global write "Meas_global.vi" "Ch & spans"(w498) -> ()
          }
          frame #17 {
            w548 = u8 0  # Disabled
            n258 = local read "Read Setup File?"() -> (w545:bool)
            n259 = global read "Meas_global.vi" "Acquisition vi to Run"() -> (w544:string)
            n260 = Equal?(x=w551, y=Post_Process."Take New Data" ("Post Process")) -> (x = y?=w550:bool)
            n261 = Equal?(x="ADAM_Server_Channels.vi", y=w544) -> (x = y?=w542:bool)
            n262 = And(x=w545, y=w542) -> (x .and. y?=w554:bool)
            n263 = Or(x="Select ADAM Channels", y=w554) -> (x .or. y?=w549:bool)
            n264 = And(x=w550, y=w549) -> (x .and. y?=w538:bool)
            n265 = case shown="True" w538 {
              tunnel: [w555 w556] -> w539
              tunnel: w540 -> [w555 w559]
              tunnel: "Select ADAM Channels" -> [_ w558]
              tunnel: w542 -> [_ w557]
              frame False {
              }
              frame True {
                n266 = stacked-sequence {
                  seq-local: [w561 _ _] -> [_ w571 _]
                  tunnel: w559 -> [w563 w570 _]
                  tunnel: [_ w568 _] -> w556
                  tunnel: w558 -> [w565 _ w577]
                  tunnel: w557 -> [w564 _ _]
                  frame #0 {
                    n267 = Not(x=w564) -> (.not. x?=w560:bool)
                    n268 = Array Size(array=w563) -> ()  [unwired: 1 out]
                    n269 = for {
                      tunnel: w563 -> [w567] mode=indexing
                      tunnel: [w566] -> w562 mode=indexing
                      n270 = Unbundle By Name(w567) -> ("Ch Name"=w566:string)
                    }
                    n271 = call "Get_local_ADAM_Chs.vi"("Local ADAM?"=w560, "Show setup"=w565, "Desired Local ADAM Channels"=w562) -> ("Choosen Channels"=w561:string[])  [unwired: 1 out]
                  }
                  frame #1 {
                    n272 = for {
                      tunnel: [w576] -> w568 mode=indexing
                      tunnel: w571 -> [w575] mode=indexing
                      tunnel: w570 -> [w574]
                      i -> [w573]
                      n273 = Index Array(array=w574, index=w573) -> (element=w572:T20)
                      n274 = Bundle By Name(cluster=w572, "Ch No"=w573, "Ch Name"=w575) -> (w576:T20)
                    }
                    n275 = Array Size(array=w568) -> (size(s)=w569:i32)
                    n276 = local write "No of Analogue inst"(w569) -> ()
                  }
                  frame #2 {
                    n277 = case shown="True" w577 {
                      frame False {
                      }
                      frame True {
                        n278 = local write "Select ADAM Channels"(FALSE ("Select Local ADAM Channels")) -> ()
                      }
                    }
                  }
                }
              }
            }
            n279 = Select(t=w548, s=w542, f=u8 2 ("Disabled")) -> (s? t:f=w546:u8)
            n280 = property on="Ch Name" class="Str"("Visible"=w542) -> ()  [unwired: 2 in, 2 out]
            n281 = property on="Select ADAM Channels" class="Bool (strict)"("Disabled"=w546) -> ()  [unwired: 2 in, 2 out]
            n282 = Not(x=w542) -> (.not. x?=w541:bool)
            n283 = property on="high limit" class="DigNum (strict)"("Visible"=w541) -> ()  [unwired: 2 in, 2 out]
            n284 = property on="low limit" class="DigNum (strict)"("Visible"=w541) -> ()  [unwired: 2 in, 2 out]
            n285 = property on="Ch No" class="DigNum (strict)"("Visible"=w541) -> ()  [unwired: 2 in, 2 out]
          }
          frame #18 {
            n286 = Not Equal?(x=w579, y=w580) -> (x != y?=w581:bool)
            n287 = case shown="True" w581 {
              tunnel: w580 -> [_ w582]
              frame False {
              }
              frame True {
                n288 = local write "Ch & spans choices"(w582) -> ()
              }
            }
          }
          frame #19 {
            n289 = global read "Meas_global.vi" "Duplicate channels"() -> (w584:i32[])
            n290 = case shown="True" "Select Duplicate Channels" {
              tunnel: w587 -> [_ _]
              tunnel: w585 -> [w595 w618]
              tunnel: w584 -> [w589 w611]
              tunnel: [w588 w610] -> w583
              frame False {
                n291 = for {
                  tunnel: w595 -> [w609] mode=indexing
                  tunnel: [w608] -> w596 mode=indexing
                  n292 = Unbundle By Name(w609) -> ("Inst type"=w608:T2)
                }
                n293 = for {
                  tunnel: w589 -> [w605] mode=indexing
                  tunnel: w596 -> [w607]
                  tunnel: [w606] -> w600 mode=indexing
                  tunnel: [w605] -> w597 mode=indexing
                  n294 = Index Array(array=w607, index=w605) -> (element=w606:T2)
                }
                n295 = Array Size(array=w595) -> (size(s)=w598:i32)
                n296 = Array Max & Min(array=w600) -> (max value=w601:T2, min value=w602:T2)  [unwired: 2 out]
                n297 = Array Max & Min(array=w597) -> (max index (indices)=w599:i32)  [unwired: 3 out]
                n298 = Array Size(array=w589) -> (size(s)=w594:i32)
                n299 = Equal?(x=w601, y=w602) -> (x = y?=w604:bool)
                n300 = Greater?(x=w594, y=1) -> (0:w591:bool)
                n301 = Greater?(x=w598, y=w599) -> (0:w603:bool)
                n302 = Compound Arithmetic op=AND(w591, w604, w603) -> (w590:bool)
                n303 = Select(t=w589, s=w590, f=i32[] [] ("32bit integer")) -> (s? t:f=w588:i32[])
              }
              frame True {
                n304 = for {
                  tunnel: w618 -> [w625] mode=indexing
                  shift-right: [w620] -> w614
                  shift-left: string[] [] -> [w621]
                  tunnel: w611 -> [w623]
                  tunnel: [w619] -> w613 mode=indexing
                  i -> [w624]
                  n305 = Unbundle By Name(w625) -> ("Inst name"=w619:string)
                  n306 = Search 1D Array(1D array=w623, element=w624) -> (index of element=w622:i32)  [unwired: 1 out]
                  n307 = case shown="0, Default" w622 {
                    tunnel: w621 -> [w628 w629]
                    tunnel: w619 -> [w627 _]
                    tunnel: [w626 w629] -> w620
                    frame 0, Default {
                      n308 = Build Array (concatenate)(w628, w627) -> (w626:string[])
                    }
                    frame -1 {
                    }
                  }
                }
                n309 = call "Select_Strings.vi"("Available Ch names"=w613, "Message"="Please select similar instruments whose results columns will be combined", "Selector mode"=T15."Zero or more", "Desired Ch names (in)"=w614) -> ("Ch Indicies Choosen"=w610:i32[])  [unwired: 4 out]
                n310 = local write "Select Duplicate Channels"(FALSE ("Select Local ADAM Channels")) -> ()
              }
            }
            n311 = global write "Meas_global.vi" "Duplicate channels"(w583) -> ()
          }
          frame #20 {
            n312 = local read "XW Present?"() -> (w632:bool)
            n313 = case shown="\"Take LDA data\"" "LDA data" {
              tunnel: [w641 w644] -> w634
              tunnel: w635 -> [_ w642]
              tunnel: w636 -> [_ _]
              tunnel: [w641 w643] -> w631
              frame "No LDA data" {
                w640 = FALSE  # Synchronise Analogue channels with LDA
                w641 = u8 2  # Disabled
                n314 = local write "Synchronise Analogue channels with LDA"(w640) -> ()
              }
              frame "Take LDA data" {
                n315 = stacked-sequence {
                  tunnel: [w645 _] -> w644
                  tunnel: [_ w647] -> w643
                  tunnel: w642 -> [_ w648]
                  frame #0 {
                    w645 = u8 0  # Disabled
                  }
                  frame #1 {
                    n316 = Array Size(array=w648) -> (size(s)=w649:i32)
                    n317 = Not Equal To 0?(x=w649) -> (x != 0?=w646:bool)
                    n318 = case shown="False" w646 {
                      tunnel: w646 -> [w651 _]
                      tunnel: [w650 w652] -> w647
                      frame False {
                        w650 = u8 2  # Disabled
                        n319 = local write "Synchronise Analogue channels with LDA"(w651) -> ()
                      }
                      frame True {
                        w652 = u8 0  # Disabled
                      }
                    }
                  }
                }
              }
            }
            n320 = property on="Cross wire/LDA" class="Enum (strict)"("Visible"=w632) -> ()  [unwired: 2 in, 2 out]
            n321 = case shown="True" w632 {
              tunnel: [w638 "Cross wire"] -> w630
              frame False {
                w638 = T7."2nd component as calculated"  # Cross wire/LDA
              }
              frame True {
              }
            }
            n322 = global write "Meas_global.vi" "Cross wire + or -ve"(w630) -> ()
            n323 = Wait (ms)(milliseconds to wait=u32 100) -> ()  [unwired: 1 out]
            n324 = property on="Synchronise Analogue channels with LDA" class="Bool (strict)"("Disabled"=w631) -> ()  [unwired: 2 in, 2 out]
            n325 = property on="LDA set up" class="Clust (strict)"("Disabled"=w634) -> ()  [unwired: 2 in, 2 out]
          }
          frame #21 {
            n326 = And(x=w658, y=w659) -> (x .and. y?=w657:bool)
            n327 = local read "Synchronise Analogue channels with LDA"() -> (w656:bool)
            n328 = while {
              shift-left: _ -> [w685]
              shift-right: [w686] -> w653
              tunnel: [w687] -> w655
              stop <- FALSE continue-if-true
              n329 = local read "Setup filename selector"() -> (w686:u16)
              n330 = Not Equal?(x=w686, y=w685) -> (x != y?=w687:bool)
            }
            n331 = case shown="True" w656 {
              tunnel: w660 -> [_ w671]
              tunnel: w657 -> [_ w670]
              frame False {
              }
              frame True {
                n332 = case shown="True" w670 {
                  tunnel: w671 -> [_ w674]
                  frame False {
                  }
                  frame True {
                    n333 = for {
                      tunnel: w674 -> [w683] mode=indexing
                      tunnel: [w676] -> w673 mode=indexing
                      n334 = Unbundle By Name(w683) -> ("Inst type"=w682:T2, "Symbol"=w680:string)
                      n335 = Equal?(x=w680, y="Sync") -> (x = y?=w678:bool)
                      n336 = Equal?(x=Inst_type."Raw voltage" ("Inst type"), y=w682) -> (x = y?=w677:bool)
                      n337 = And(x=w677, y=w678) -> (x .and. y?=w676:bool)
                    }
                    n338 = Or Array Elements(Boolean array=w673) -> (logical OR=w672:bool)
                    n339 = case shown="False" w672 {
                      frame False {
                        n340 = One Button Dialog(message="To Perform LDA Sync you must provide a Raw voltage channel having the symbol \"Sync\"") -> ()  [unwired: 2 out]
                      }
                      frame True {
                      }
                    }
                  }
                }
              }
            }
            n341 = case shown="True" w655 {
              tunnel: [FALSE ("exists?") w669] -> w654
              tunnel: w653 -> [_ w667]
              frame False {
              }
              frame True {
                n342 = local read "Setup Paths"() -> (w668:string[])
                n343 = Index Array(array=w668, index=w667) -> (element=w665:string)
                n344 = call "Setup_Filepath.vi"("Setup File Type"=Setup_Filetype."Measurement Setups", "Filename in"=w665) -> ("Filename Out"=w664:path)  [unwired: 1 out]
                n345 = call "Does_file_exist_(simple).vi"("Pathname"=w664) -> ("exists?"=w669:bool)
              }
            }
            n346 = local write "Read Setup File?"(w654) -> ()
            n347 = Current VI's Path() -> (path=w661:path)
            n348 = call "Close_Panel_and_Abort.vi"("Vi path"=w661, "stop"="stop") -> ()  [unwired: 1 out]
          }
        }
      }
    }
    frame #5 {
      n349 = local read "LDA data"() -> (w690:enum16{"No LDA data", "Take LDA data"})
      n350 = case shown="\"Take LDA data\"" w690 {
        tunnel: [FALSE ("Synchronise Analogue channels with LDA") "Synchronise Analogue channels with LDA"] -> w689
        frame "No LDA data" {
        }
        frame "Take LDA data" {
        }
      }
      n351 = global write "Meas_global.vi" "Synchronise with LDA"(w689) -> ()
      n352 = global write "Meas_global.vi" "LDA data"(w690) -> ()
      n353 = global write "Meas_global.vi" "LDA set up"("LDA set up") -> ()
    }
    frame #6 {
      n354 = stacked-sequence {
        seq-local: [_ w730 _ _] -> [_ _ _ w788]
        seq-local: [_ _ w756 _] -> [_ _ _ w787]
        seq-local: [w698 _ _ _] -> [_ _ _ w775]
        tunnel: w695 -> [w697 _ _ w779]
        tunnel: w694 -> [_ _ _ w778]
        tunnel: w693 -> [w696 _ _ _]
        frame #0 {
          n355 = local read "PWA Data"() -> (w699:T1)
          n356 = case shown="\"One Ch PWA\"" w699 {
            tunnel: ["" w708] -> w698
            tunnel: w697 -> [_ w707]
            tunnel: w696 -> [_ w703]
            frame "No PWA Data" {
            }
            frame "One Ch PWA" {
              n357 = Not Equal?(x="Calib_Setup.xls", y=w703) -> (x != y?=w702:bool)
              n358 = case shown="\"Setup Front Panel\"" w707 {
                tunnel: [w712 w715 w718 w721] -> w706
                tunnel: [w711 w714 w717 w720] -> w705
                tunnel: [w710 w713 w716 w719] -> w701
                tunnel: w702 -> [w710 w713 w716 _]
                frame "Show Setup" {
                  w712 = TRUE  # Show Panel?
                  w711 = T4 FALSE  # OK
                }
                frame "Run Program" {
                  w715 = FALSE  # Show Panel?
                  w714 = T4 TRUE  # OK
                }
                frame "Save Current Setup" {
                  w718 = FALSE  # Show Panel?
                  w717 = T4 TRUE  # OK
                }
                frame "Setup Front Panel" {
                  w719 = FALSE  # Check Calib file?
                  w721 = FALSE  # Show Panel?
                  w720 = T4 TRUE  # OK
                }
              }
              n359 = global read "Meas_global.vi" "Pre Setup String"() -> (w709:string)
              n360 = call "PWA_Setup_Panel.vi"("Show Panel?"=w706, "Check Calib file?"=w701, "OK"=w705, "Incoming Setup String"=w709) -> ("Outgoing Setup String"=w708:string)  [unwired: 3 out]
            }
          }
        }
        frame #1 {
          n361 = local read "LDA set up"() -> (w735:T6)
          n362 = global read "Meas_global.vi" "Duplicate channels"() -> (w734:i32[])
          n363 = Unbundle By Name(w735) -> ("dimensions"=w727:enum16{"1D", "2D"}, "Analogue Freq Multiplier"=w725:dbl)
          n364 = case shown="\"2D\"" w727 {
            tunnel: ["1D" "2D"] -> w729
            frame "1D" {
            }
            frame "2D" {
            }
          }
          n365 = for {
            shift-right: [w738] -> w732
            shift-left: "" -> [w741]
            tunnel: w734 -> [w742] mode=indexing
            n366 = Number To Decimal String(number=w742) -> (decimal integer string=w740:string)  [unwired: 1 out]
            n367 = Concatenate Strings(w741, w740, "; ") -> (w738:string)
          }
          n368 = call "Characters_to_string.vi"("Characters to write"=w729, "Label for characters"="LDA Dimensions") -> ("Output string"=w728:string)
          n369 = call "Value_to_string.vi"("Value"=w725, "Label for value"="LDA Analog Freq Multiplier") -> ("Output string"=w722:string)  [unwired: 1 in]
          n370 = call "Characters_to_string.vi"("Characters to write"=w732, "Label for characters"="Log_Similar_Measurements_in_the _same_column") -> ("Output string"=w723:string)
          n371 = Concatenate Strings(w728, w722, w723) -> (w730:string)
        }
        frame #2 {
          n372 = global write "Meas_global.vi" "Trigger mode"("Trigger mode") -> ()
          n373 = local read "Cross wire"() -> (w759:T7)
          n374 = global read "Preference_global.vi" "Rig Setup"() -> (w745:string)
          n375 = Match Pattern(string=w745, regular expression="-") -> (before substring=w744:string)  [unwired: 4 out]
          n376 = case shown="\"Free Running\"" "Trigger mode" {
            tunnel: ["Free Running" "Trigger Every Block" "Trigger Every Sample" "Start on Trigger"] -> w754
            frame "Free Running" {
            }
            frame "Trigger Every Block" {
            }
            frame "Trigger Every Sample" {
            }
            frame "Start on Trigger" {
            }
          }
          n377 = property on="PWA Data" class="Enum (strict)"() -> ("Strings []"=w750:string[])  [unwired: 2 in, 2 out]
          n378 = global write "Meas_global.vi" "PWA Data"("PWA Data") -> ()
          n379 = Equal?(x=T7."2nd component multipled by -1" ("Cross wire/LDA"), y=w759) -> (x = y?=w758:bool)
          n380 = case shown="\"EnFlo_Tunnel\"" w744 {
            tunnel: ["" w766] -> w743
            frame "False", Default {
            }
            frame "EnFlo_Tunnel" {
              n381 = call "Characters_to_string.vi"("Characters to write"="FALSE", "Label for characters"="Show_all_EnFlo_Tunnel_Columns") -> ("Output string"=w766:string)
            }
          }
          n382 = Index Array(array=w750, index="PWA Data") -> (element=w749:string)
          n383 = Select(t="TRUE", s=w758, f="FALSE") -> (s? t:f=w761:string)
          n384 = call "Characters_to_string.vi"("Characters to write"=w749, "Label for characters"="Pulsed_Wire_Data" ("Variable name")) -> ("Output string"=w748:string)
          n385 = call "Characters_to_string.vi"("Characters to write"=w761, "Label for characters"="Invert Second Component") -> ("Output string"=w757:string)
          n386 = call "Characters_to_string.vi"("Characters to write"=w754, "Label for characters"="Trigger mode") -> ("Output string"=w752:string)
          n387 = Concatenate Strings(w752, w748, w757, w743) -> (w756:string)
        }
        frame #3 {
          w780 = FALSE  # Show Panel?
          n388 = for {
            tunnel: w778 -> [w793] mode=indexing
            tunnel: [w792] -> w774 mode=indexing
            n389 = Unbundle By Name(w793) -> ("Ch Name"=w792:string)
          }
          n390 = global read "Meas_global.vi" "Pre Setup String"() -> (w781:string)
          n391 = call "Choose_Plug_In_to_Run.vi"("setup"=w779, "Show Panel?"=w780, "Setup String In"=w781) -> ("Setup String Out"=w782:string)  [unwired: 1 out]
          n392 = Array To Spreadsheet String(array=w774, 3:"%s" ("format string")) -> (spreadsheet string=w776:string)  [unwired: 1 out]
          n393 = call "Add_label_to_string.vi"("String to write"=w776, "File Label"="Local ADAM Channels") -> ("Output string"=w789:string)
          n394 = call "Date_and_Time_to_string.vi"() -> ("Date and time (spreadsheet)"=w784:string)
          n395 = global read "Meas_global.vi" "New Setup String"() -> (w783:string)
          n396 = call "Value_to_string.vi"("Value"="Sync Delay Time (ms)", "Label for value"="Sync Delay Time (ms)" ("Label for characters")) -> ("Output string"=w777:string)  [unwired: 1 in]
          n397 = Concatenate Strings(w783, w775, w782, w784, w788, w787, w789, w777) -> (w791:string)
          n398 = global write "Meas_global.vi" "New Setup String"(w791) -> ()
          n399 = global write "LDA_meas_global_1.vi" "Sync Delay Time (ms)"("Sync Delay Time (ms)") -> ()
        }
      }
    }
    frame #7 {
      n400 = case shown="\"Post Process Raw Data File\"" w796 {
        tunnel: w795 -> [w803 w838]
        tunnel: [w797 w832] -> w794
        frame "Take New Data" {
          n401 = for {
            tunnel: w803 -> [w814] mode=indexing
            shift-right: [w810] -> w800
            shift-left: i16[] [] -> [w812]
            shift-right: [w808] -> w799
            shift-left: path[] [] -> [w809]
            tunnel: [w805] -> w797 mode=indexing
            n402 = Unbundle By Name(w814) -> ("Use Latest"=w807:bool, "Inst type"=w813:T2, "Ch No"=w811:i16, "Calib filename"=w806:path)
            n403 = call "Current_Filepath.vi"("Filename in"=w806, "Data Type"="Calibrations") -> ("Filename Out"=w805:path)  [unwired: 1 out]
            n404 = case shown="\"Propeller anemometer\", Default" w813 {
              tunnel: w812 -> [w821 w831]
              tunnel: w811 -> [w820 _]
              tunnel: [w819 w831] -> w810
              tunnel: w809 -> [w818 w830]
              tunnel: w806 -> [w817 _]
              tunnel: [w816 w830] -> w808
              tunnel: w807 -> [w815 _]
              frame "Propeller anemometer", Default {
                n405 = case shown="False" w815 {
                  tunnel: w821 -> [w827 w829]
                  tunnel: w820 -> [w826 _]
                  tunnel: [w825 w829] -> w819
                  tunnel: w818 -> [w824 w828]
                  tunnel: w817 -> [w823 _]
                  tunnel: [w822 w828] -> w816
                  frame False {
                    n406 = Build Array (concatenate)(w827, w826) -> (w825:i16[])
                    n407 = Build Array (concatenate)(w824, w823) -> (w822:path[])
                  }
                  frame True {
                  }
                }
              }
              frame "Raw voltage" {
              }
            }
          }
          n408 = call "Current_Calib_Filenames.vi"("Calib Filename"=w799, "Channel Numbers"=w800, "Mode"=App_Global."Write to Global") -> ()  [unwired: 3 out]
        }
        frame "Post Process Raw Data File" {
          n409 = for {
            tunnel: w838 -> [w844] mode=indexing
            tunnel: [w843] -> w832 mode=indexing
            n410 = Unbundle By Name(w844) -> ("Calib filename"=w843:path)
          }
          n411 = global read "Meas_global.vi" "Pre Setup String"() -> (w837:string)
          n412 = call "Get_Characters_from_string.vi"("Input string"=w837, "Variable name"="Skip_Block_Numbers_(eg 1;2;5;12)") -> ("Status"=w835:enum16{"Char in string", "Char not in string"}, "Value"=w834:string)  [unwired: 1 in]
          n413 = case shown="\"Char in string\"" w835 {
            tunnel: w834 -> [w841 _]
            tunnel: [w839 i32[] []] -> w833
            frame "Char in string" {
              n414 = call "Get_array_values_fr_String.vi"("String Value"=w841) -> ("Numeric Array"=w840:dbl[])  [unwired: 1 out]
              n415 = To Long Integer(number=w840) -> (32bit integer=w839:i32[])
            }
            frame "Char not in string" {
            }
          }
          n416 = global write "Meas_global.vi" "Blocks to Skip"(w833) -> ()
        }
      }
    }
    frame #8 {
      n417 = global read "Meas_global.vi" "Pre Setup String"() -> (w845:string)
      n418 = for {
        tunnel: [w856] -> w848 mode=indexing
        tunnel: w847 -> [w853] mode=indexing
        tunnel: w846 -> [w855] mode=indexing
        tunnel: w845 -> [w854]
        n419 = Unbundle By Name(w853) -> ("Code name"=w852:string)
        n420 = Concatenate Strings(w852, "_Av_SamplingRate" ("string")) -> (w850:string)
        n421 = call "Get_value_from_string.vi"("Input string"=w854, "Variable name"=w850) -> ("Value"=w849:dbl)  [unwired: 1 in, 1 out]
        n422 = Bundle By Name(cluster=w853, "Calib File"=w855, "Av Sampling Rate"=w849) -> (w856:T8)
      }
      "Analysis Info cluster" <- w848
    }
  }
